vi "GenerateHistogramIndices.vi"(7 "Last laser in":bool, 11 "Laser in":bool[](array[boolean])=[FALSE, FALSE, FALSE, FALSE, FALSE, FALSE, FALSE, FALSE, FALSE, FALSE, FALSE, FALSE, FALSE, FALSE, FALSE, FALSE, FALSE, FALSE, FALSE, FALSE, FALSE, FALSE, FALSE, FALSE, FALSE, FALSE, FALSE, FALSE, FALSE, FALSE, FALSE, FALSE, FALSE, FALSE, FALSE, FALSE, FALSE, FALSE, FALSE, FALSE, FALSE, FALSE, FALSE, FALSE, FALSE, FALSE, FALSE, FALSE, FALSE, FALSE, FALSE, FALSE, FALSE, FALSE, FALSE, FALSE, FALSE, FALSE, FALSE, FALSE]) -> (3 "Index array out":i32[](array[numeric]), 5 "Last laser out":bool)   [LabVIEW 2012]
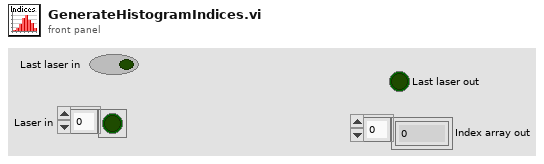
[diagram p1: front panel]
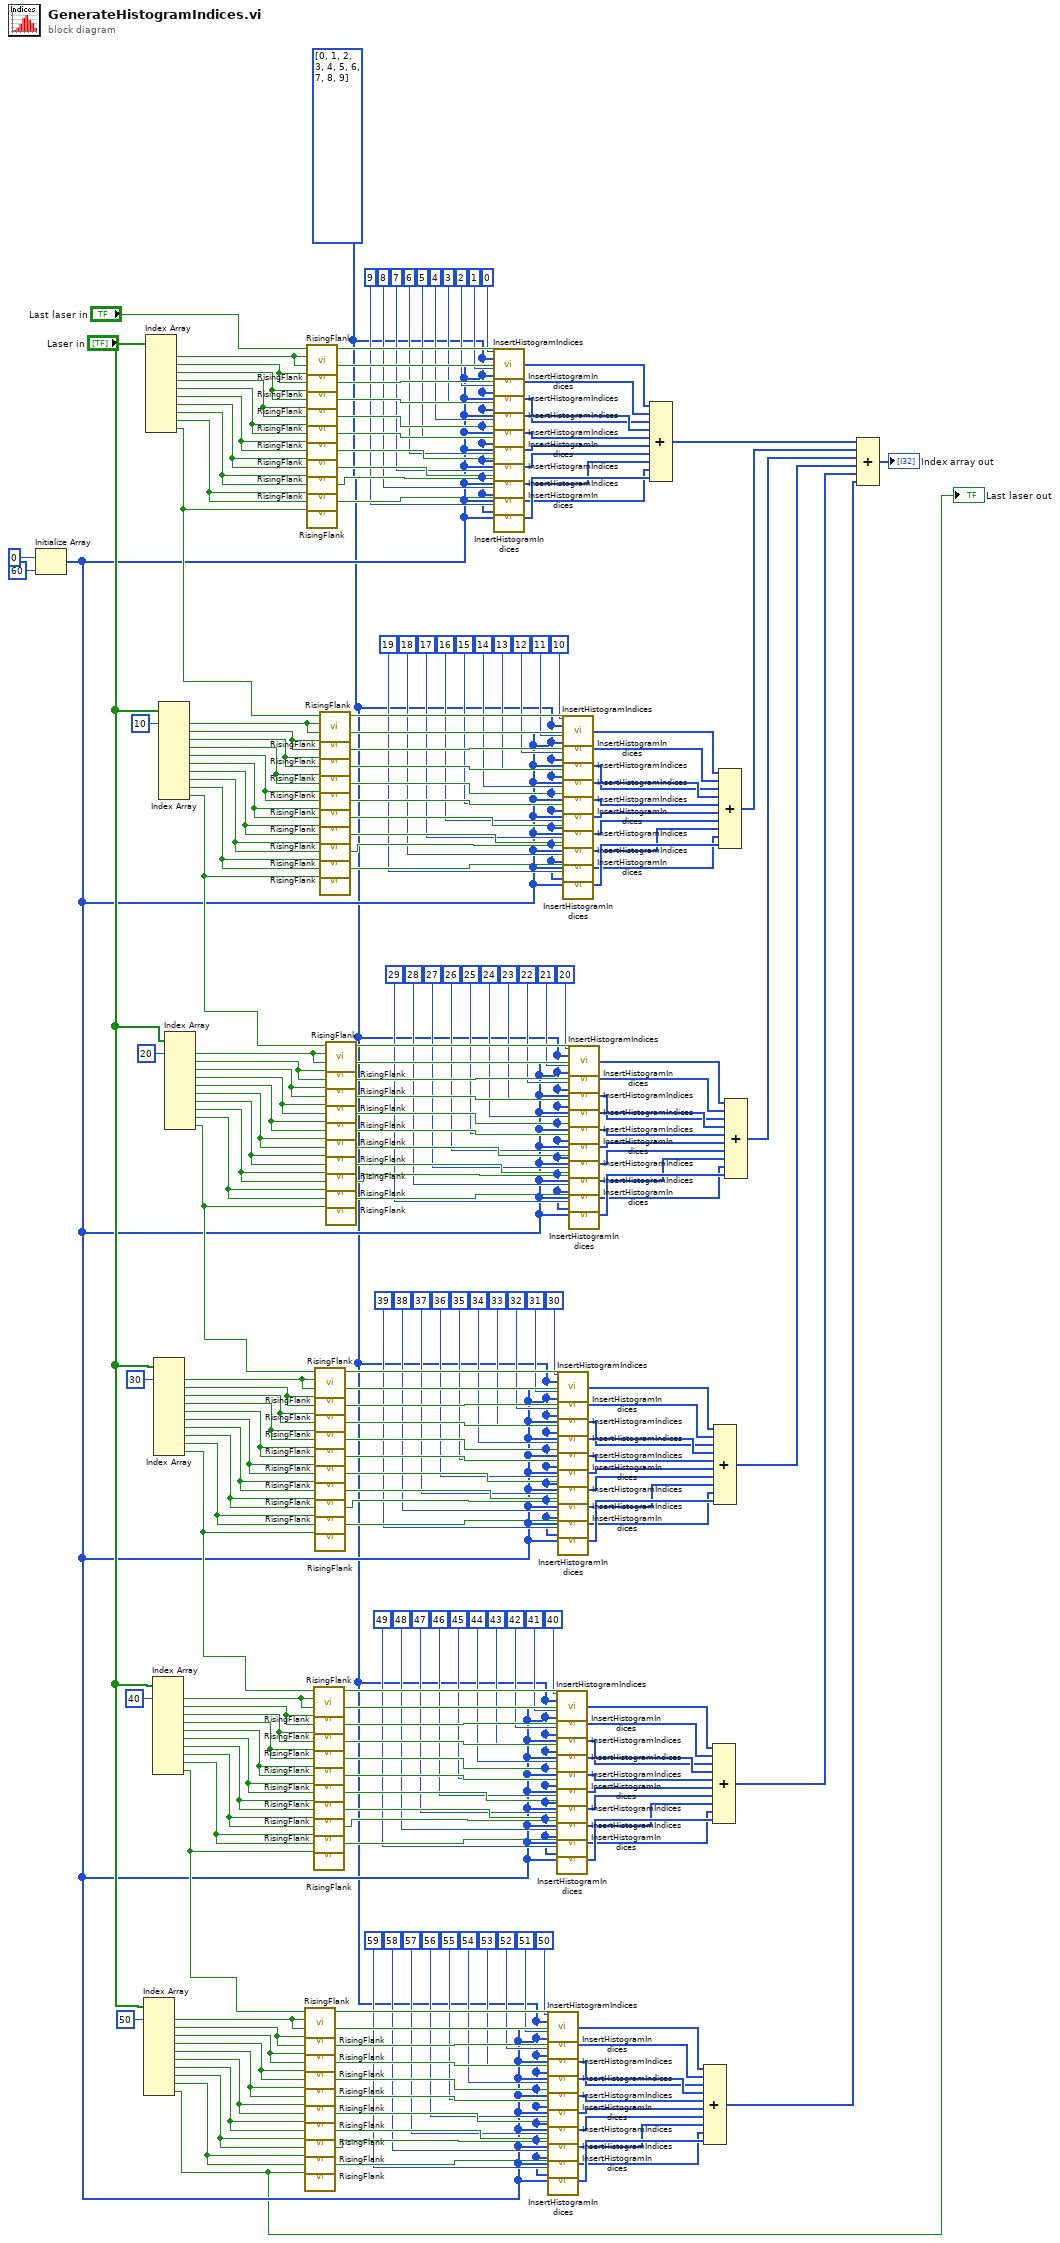
[diagram p0: block diagram]
diagram:
  w9 = i32[] [0, 1, 2, 3, 4, 5, 6, 7, 8, 9]
  n1 = Initialize Array(0, 60 ("dimension size")) -> (w10:i32[])
  n2 = Index Array(array="Laser in", index #1=50 ("index")) -> (element #1=w52:bool, element #2=w49:bool, element #3=w48:bool, element #4=w47:bool, element #5=w46:bool, element #6=w45:bool, element #7=w44:bool, element #8=w43:bool, element #9=w42:bool, element #10=w1:bool)  [unwired: 9 in]
  "Last laser out" <- w1
  n3 = Index Array(array="Laser in") -> (element #1=w255:bool, element #2=w252:bool, element #3=w251:bool, element #4=w250:bool, element #5=w249:bool, element #6=w248:bool, element #7=w247:bool, element #8=w246:bool, element #9=w245:bool, element #10=w176:bool)  [unwired: 10 in]
  n4 = Index Array(array="Laser in", index #1=40 ("index")) -> (element #1=w93:bool, element #2=w90:bool, element #3=w89:bool, element #4=w88:bool, element #5=w87:bool, element #6=w86:bool, element #7=w85:bool, element #8=w84:bool, element #9=w83:bool, element #10=w11:bool)  [unwired: 9 in]
  n5 = Index Array(array="Laser in", index #1=30 ("index")) -> (element #1=w134:bool, element #2=w131:bool, element #3=w130:bool, element #4=w129:bool, element #5=w128:bool, element #6=w127:bool, element #7=w126:bool, element #8=w125:bool, element #9=w124:bool, element #10=w53:bool)  [unwired: 9 in]
  n6 = Index Array(array="Laser in", index #1=10 ("index")) -> (element #1=w216:bool, element #2=w213:bool, element #3=w212:bool, element #4=w211:bool, element #5=w210:bool, element #6=w209:bool, element #7=w208:bool, element #8=w207:bool, element #9=w206:bool, element #10=w135:bool)  [unwired: 9 in]
  n7 = Index Array(array="Laser in", index #1=20 ("index")) -> (element #1=w175:bool, element #2=w172:bool, element #3=w171:bool, element #4=w170:bool, element #5=w169:bool, element #6=w168:bool, element #7=w167:bool, element #8=w166:bool, element #9=w165:bool, element #10=w94:bool)  [unwired: 9 in]
  n8 = call "RisingFlank.vi"("2nd sample"=w52, "1st sample"=w11) -> ("Rising flank?"=w51:bool)  [unwired: 7 in]
  n9 = call "RisingFlank.vi"("2nd sample"=w49, "1st sample"=w52) -> ("Rising flank?"=w50:bool)  [unwired: 7 in]
  n10 = call "RisingFlank.vi"("2nd sample"=w48, "1st sample"=w49) -> ("Rising flank?"=w41:bool)  [unwired: 7 in]
  n11 = call "RisingFlank.vi"("2nd sample"=w47, "1st sample"=w48) -> ("Rising flank?"=w40:bool)  [unwired: 7 in]
  n12 = call "RisingFlank.vi"("2nd sample"=w46, "1st sample"=w47) -> ("Rising flank?"=w39:bool)  [unwired: 7 in]
  n13 = call "RisingFlank.vi"("2nd sample"=w45, "1st sample"=w46) -> ("Rising flank?"=w38:bool)  [unwired: 7 in]
  n14 = call "RisingFlank.vi"("2nd sample"=w44, "1st sample"=w45) -> ("Rising flank?"=w37:bool)  [unwired: 7 in]
  n15 = call "RisingFlank.vi"("2nd sample"=w43, "1st sample"=w44) -> ("Rising flank?"=w36:bool)  [unwired: 7 in]
  n16 = call "RisingFlank.vi"("2nd sample"=w42, "1st sample"=w43) -> ("Rising flank?"=w35:bool)  [unwired: 7 in]
  n17 = call "RisingFlank.vi"("2nd sample"=w1, "1st sample"=w42) -> ("Rising flank?"=w34:bool)  [unwired: 7 in]
  n18 = call "RisingFlank.vi"("2nd sample"=w255, "1st sample"="Last laser in") -> ("Rising flank?"=w254:bool)  [unwired: 7 in]
  n19 = call "RisingFlank.vi"("2nd sample"=w252, "1st sample"=w255) -> ("Rising flank?"=w253:bool)  [unwired: 7 in]
  n20 = call "RisingFlank.vi"("2nd sample"=w251, "1st sample"=w252) -> ("Rising flank?"=w244:bool)  [unwired: 7 in]
  n21 = call "RisingFlank.vi"("2nd sample"=w250, "1st sample"=w251) -> ("Rising flank?"=w243:bool)  [unwired: 7 in]
  n22 = call "RisingFlank.vi"("2nd sample"=w249, "1st sample"=w250) -> ("Rising flank?"=w242:bool)  [unwired: 7 in]
  n23 = call "RisingFlank.vi"("2nd sample"=w248, "1st sample"=w249) -> ("Rising flank?"=w241:bool)  [unwired: 7 in]
  n24 = call "RisingFlank.vi"("2nd sample"=w247, "1st sample"=w248) -> ("Rising flank?"=w240:bool)  [unwired: 7 in]
  n25 = call "RisingFlank.vi"("2nd sample"=w246, "1st sample"=w247) -> ("Rising flank?"=w239:bool)  [unwired: 7 in]
  n26 = call "RisingFlank.vi"("2nd sample"=w245, "1st sample"=w246) -> ("Rising flank?"=w238:bool)  [unwired: 7 in]
  n27 = call "RisingFlank.vi"("2nd sample"=w176, "1st sample"=w245) -> ("Rising flank?"=w237:bool)  [unwired: 7 in]
  n28 = call "RisingFlank.vi"("2nd sample"=w93, "1st sample"=w53) -> ("Rising flank?"=w92:bool)  [unwired: 7 in]
  n29 = call "RisingFlank.vi"("2nd sample"=w90, "1st sample"=w93) -> ("Rising flank?"=w91:bool)  [unwired: 7 in]
  n30 = call "RisingFlank.vi"("2nd sample"=w89, "1st sample"=w90) -> ("Rising flank?"=w82:bool)  [unwired: 7 in]
  n31 = call "RisingFlank.vi"("2nd sample"=w88, "1st sample"=w89) -> ("Rising flank?"=w81:bool)  [unwired: 7 in]
  n32 = call "RisingFlank.vi"("2nd sample"=w87, "1st sample"=w88) -> ("Rising flank?"=w80:bool)  [unwired: 7 in]
  n33 = call "RisingFlank.vi"("2nd sample"=w86, "1st sample"=w87) -> ("Rising flank?"=w79:bool)  [unwired: 7 in]
  n34 = call "RisingFlank.vi"("2nd sample"=w85, "1st sample"=w86) -> ("Rising flank?"=w78:bool)  [unwired: 7 in]
  n35 = call "RisingFlank.vi"("2nd sample"=w84, "1st sample"=w85) -> ("Rising flank?"=w77:bool)  [unwired: 7 in]
  n36 = call "RisingFlank.vi"("2nd sample"=w83, "1st sample"=w84) -> ("Rising flank?"=w76:bool)  [unwired: 7 in]
  n37 = call "RisingFlank.vi"("2nd sample"=w11, "1st sample"=w83) -> ("Rising flank?"=w75:bool)  [unwired: 7 in]
  n38 = call "RisingFlank.vi"("2nd sample"=w134, "1st sample"=w94) -> ("Rising flank?"=w133:bool)  [unwired: 7 in]
  n39 = call "RisingFlank.vi"("2nd sample"=w131, "1st sample"=w134) -> ("Rising flank?"=w132:bool)  [unwired: 7 in]
  n40 = call "RisingFlank.vi"("2nd sample"=w130, "1st sample"=w131) -> ("Rising flank?"=w123:bool)  [unwired: 7 in]
  n41 = call "RisingFlank.vi"("2nd sample"=w129, "1st sample"=w130) -> ("Rising flank?"=w122:bool)  [unwired: 7 in]
  n42 = call "RisingFlank.vi"("2nd sample"=w128, "1st sample"=w129) -> ("Rising flank?"=w121:bool)  [unwired: 7 in]
  n43 = call "RisingFlank.vi"("2nd sample"=w127, "1st sample"=w128) -> ("Rising flank?"=w120:bool)  [unwired: 7 in]
  n44 = call "RisingFlank.vi"("2nd sample"=w126, "1st sample"=w127) -> ("Rising flank?"=w119:bool)  [unwired: 7 in]
  n45 = call "RisingFlank.vi"("2nd sample"=w125, "1st sample"=w126) -> ("Rising flank?"=w118:bool)  [unwired: 7 in]
  n46 = call "RisingFlank.vi"("2nd sample"=w124, "1st sample"=w125) -> ("Rising flank?"=w117:bool)  [unwired: 7 in]
  n47 = call "RisingFlank.vi"("2nd sample"=w53, "1st sample"=w124) -> ("Rising flank?"=w116:bool)  [unwired: 7 in]
  n48 = call "RisingFlank.vi"("2nd sample"=w216, "1st sample"=w176) -> ("Rising flank?"=w215:bool)  [unwired: 7 in]
  n49 = call "RisingFlank.vi"("2nd sample"=w213, "1st sample"=w216) -> ("Rising flank?"=w214:bool)  [unwired: 7 in]
  n50 = call "RisingFlank.vi"("2nd sample"=w212, "1st sample"=w213) -> ("Rising flank?"=w205:bool)  [unwired: 7 in]
  n51 = call "RisingFlank.vi"("2nd sample"=w211, "1st sample"=w212) -> ("Rising flank?"=w204:bool)  [unwired: 7 in]
  n52 = call "RisingFlank.vi"("2nd sample"=w210, "1st sample"=w211) -> ("Rising flank?"=w203:bool)  [unwired: 7 in]
  n53 = call "RisingFlank.vi"("2nd sample"=w209, "1st sample"=w210) -> ("Rising flank?"=w202:bool)  [unwired: 7 in]
  n54 = call "RisingFlank.vi"("2nd sample"=w208, "1st sample"=w209) -> ("Rising flank?"=w201:bool)  [unwired: 7 in]
  n55 = call "RisingFlank.vi"("2nd sample"=w207, "1st sample"=w208) -> ("Rising flank?"=w200:bool)  [unwired: 7 in]
  n56 = call "RisingFlank.vi"("2nd sample"=w206, "1st sample"=w207) -> ("Rising flank?"=w199:bool)  [unwired: 7 in]
  n57 = call "RisingFlank.vi"("2nd sample"=w135, "1st sample"=w206) -> ("Rising flank?"=w198:bool)  [unwired: 7 in]
  n58 = call "RisingFlank.vi"("2nd sample"=w175, "1st sample"=w135) -> ("Rising flank?"=w174:bool)  [unwired: 7 in]
  n59 = call "RisingFlank.vi"("2nd sample"=w172, "1st sample"=w175) -> ("Rising flank?"=w173:bool)  [unwired: 7 in]
  n60 = call "RisingFlank.vi"("2nd sample"=w171, "1st sample"=w172) -> ("Rising flank?"=w164:bool)  [unwired: 7 in]
  n61 = call "RisingFlank.vi"("2nd sample"=w170, "1st sample"=w171) -> ("Rising flank?"=w163:bool)  [unwired: 7 in]
  n62 = call "RisingFlank.vi"("2nd sample"=w169, "1st sample"=w170) -> ("Rising flank?"=w162:bool)  [unwired: 7 in]
  n63 = call "RisingFlank.vi"("2nd sample"=w168, "1st sample"=w169) -> ("Rising flank?"=w161:bool)  [unwired: 7 in]
  n64 = call "RisingFlank.vi"("2nd sample"=w167, "1st sample"=w168) -> ("Rising flank?"=w160:bool)  [unwired: 7 in]
  n65 = call "RisingFlank.vi"("2nd sample"=w166, "1st sample"=w167) -> ("Rising flank?"=w159:bool)  [unwired: 7 in]
  n66 = call "RisingFlank.vi"("2nd sample"=w165, "1st sample"=w166) -> ("Rising flank?"=w158:bool)  [unwired: 7 in]
  n67 = call "RisingFlank.vi"("2nd sample"=w94, "1st sample"=w165) -> ("Rising flank?"=w157:bool)  [unwired: 7 in]
  n68 = call "InsertHistogramIndices.vi"("Insert index"=0, "Rising flank?"=w254, "Histogram indices"=w9, "Master array in"=w10) -> ("Master array out"=w226:i32[])  [unwired: 11 in]
  n69 = call "InsertHistogramIndices.vi"("Insert index"=1, "Rising flank?"=w253, "Histogram indices"=w9, "Master array in"=w10) -> ("Master array out"=w225:i32[])  [unwired: 11 in]
  n70 = call "InsertHistogramIndices.vi"("Insert index"=2, "Rising flank?"=w244, "Histogram indices"=w9, "Master array in"=w10) -> ("Master array out"=w217:i32[])  [unwired: 11 in]
  n71 = call "InsertHistogramIndices.vi"("Insert index"=3, "Rising flank?"=w243, "Histogram indices"=w9, "Master array in"=w10) -> ("Master array out"=w218:i32[])  [unwired: 11 in]
  n72 = call "InsertHistogramIndices.vi"("Insert index"=4, "Rising flank?"=w242, "Histogram indices"=w9, "Master array in"=w10) -> ("Master array out"=w219:i32[])  [unwired: 11 in]
  n73 = call "InsertHistogramIndices.vi"("Insert index"=5, "Rising flank?"=w241, "Histogram indices"=w9, "Master array in"=w10) -> ("Master array out"=w220:i32[])  [unwired: 11 in]
  n74 = call "InsertHistogramIndices.vi"("Insert index"=6, "Rising flank?"=w240, "Histogram indices"=w9, "Master array in"=w10) -> ("Master array out"=w221:i32[])  [unwired: 11 in]
  n75 = call "InsertHistogramIndices.vi"("Insert index"=7, "Rising flank?"=w239, "Histogram indices"=w9, "Master array in"=w10) -> ("Master array out"=w222:i32[])  [unwired: 11 in]
  n76 = call "InsertHistogramIndices.vi"("Insert index"=8, "Rising flank?"=w238, "Histogram indices"=w9, "Master array in"=w10) -> ("Master array out"=w223:i32[])  [unwired: 11 in]
  n77 = call "InsertHistogramIndices.vi"("Insert index"=9, "Rising flank?"=w237, "Histogram indices"=w9, "Master array in"=w10) -> ("Master array out"=w224:i32[])  [unwired: 11 in]
  n78 = call "InsertHistogramIndices.vi"("Insert index"=50, "Rising flank?"=w51, "Histogram indices"=w9, "Master array in"=w10) -> ("Master array out"=w23:i32[])  [unwired: 11 in]
  n79 = call "InsertHistogramIndices.vi"("Insert index"=51, "Rising flank?"=w50, "Histogram indices"=w9, "Master array in"=w10) -> ("Master array out"=w22:i32[])  [unwired: 11 in]
  n80 = call "InsertHistogramIndices.vi"("Insert index"=52, "Rising flank?"=w41, "Histogram indices"=w9, "Master array in"=w10) -> ("Master array out"=w14:i32[])  [unwired: 11 in]
  n81 = call "InsertHistogramIndices.vi"("Insert index"=53, "Rising flank?"=w40, "Histogram indices"=w9, "Master array in"=w10) -> ("Master array out"=w15:i32[])  [unwired: 11 in]
  n82 = call "InsertHistogramIndices.vi"("Insert index"=54, "Rising flank?"=w39, "Histogram indices"=w9, "Master array in"=w10) -> ("Master array out"=w16:i32[])  [unwired: 11 in]
  n83 = call "InsertHistogramIndices.vi"("Insert index"=55, "Rising flank?"=w38, "Histogram indices"=w9, "Master array in"=w10) -> ("Master array out"=w17:i32[])  [unwired: 11 in]
  n84 = call "InsertHistogramIndices.vi"("Insert index"=56, "Rising flank?"=w37, "Histogram indices"=w9, "Master array in"=w10) -> ("Master array out"=w18:i32[])  [unwired: 11 in]
  n85 = call "InsertHistogramIndices.vi"("Insert index"=57, "Rising flank?"=w36, "Histogram indices"=w9, "Master array in"=w10) -> ("Master array out"=w19:i32[])  [unwired: 11 in]
  n86 = call "InsertHistogramIndices.vi"("Insert index"=58, "Rising flank?"=w35, "Histogram indices"=w9, "Master array in"=w10) -> ("Master array out"=w20:i32[])  [unwired: 11 in]
  n87 = call "InsertHistogramIndices.vi"("Insert index"=59, "Rising flank?"=w34, "Histogram indices"=w9, "Master array in"=w10) -> ("Master array out"=w21:i32[])  [unwired: 11 in]
  n88 = call "InsertHistogramIndices.vi"("Insert index"=40, "Rising flank?"=w92, "Histogram indices"=w9, "Master array in"=w10) -> ("Master array out"=w64:i32[])  [unwired: 11 in]
  n89 = call "InsertHistogramIndices.vi"("Insert index"=41, "Rising flank?"=w91, "Histogram indices"=w9, "Master array in"=w10) -> ("Master array out"=w63:i32[])  [unwired: 11 in]
  n90 = call "InsertHistogramIndices.vi"("Insert index"=42, "Rising flank?"=w82, "Histogram indices"=w9, "Master array in"=w10) -> ("Master array out"=w55:i32[])  [unwired: 11 in]
  n91 = call "InsertHistogramIndices.vi"("Insert index"=43, "Rising flank?"=w81, "Histogram indices"=w9, "Master array in"=w10) -> ("Master array out"=w56:i32[])  [unwired: 11 in]
  n92 = call "InsertHistogramIndices.vi"("Insert index"=44, "Rising flank?"=w80, "Histogram indices"=w9, "Master array in"=w10) -> ("Master array out"=w57:i32[])  [unwired: 11 in]
  n93 = call "InsertHistogramIndices.vi"("Insert index"=45, "Rising flank?"=w79, "Histogram indices"=w9, "Master array in"=w10) -> ("Master array out"=w58:i32[])  [unwired: 11 in]
  n94 = call "InsertHistogramIndices.vi"("Insert index"=46, "Rising flank?"=w78, "Histogram indices"=w9, "Master array in"=w10) -> ("Master array out"=w59:i32[])  [unwired: 11 in]
  n95 = call "InsertHistogramIndices.vi"("Insert index"=47, "Rising flank?"=w77, "Histogram indices"=w9, "Master array in"=w10) -> ("Master array out"=w60:i32[])  [unwired: 11 in]
  n96 = call "InsertHistogramIndices.vi"("Insert index"=48, "Rising flank?"=w76, "Histogram indices"=w9, "Master array in"=w10) -> ("Master array out"=w61:i32[])  [unwired: 11 in]
  n97 = call "InsertHistogramIndices.vi"("Insert index"=49, "Rising flank?"=w75, "Histogram indices"=w9, "Master array in"=w10) -> ("Master array out"=w62:i32[])  [unwired: 11 in]
  n98 = call "InsertHistogramIndices.vi"("Insert index"=30, "Rising flank?"=w133, "Histogram indices"=w9, "Master array in"=w10) -> ("Master array out"=w105:i32[])  [unwired: 11 in]
  n99 = call "InsertHistogramIndices.vi"("Insert index"=31, "Rising flank?"=w132, "Histogram indices"=w9, "Master array in"=w10) -> ("Master array out"=w104:i32[])  [unwired: 11 in]
  n100 = call "InsertHistogramIndices.vi"("Insert index"=32, "Rising flank?"=w123, "Histogram indices"=w9, "Master array in"=w10) -> ("Master array out"=w96:i32[])  [unwired: 11 in]
  n101 = call "InsertHistogramIndices.vi"("Insert index"=33, "Rising flank?"=w122, "Histogram indices"=w9, "Master array in"=w10) -> ("Master array out"=w97:i32[])  [unwired: 11 in]
  n102 = call "InsertHistogramIndices.vi"("Insert index"=34, "Rising flank?"=w121, "Histogram indices"=w9, "Master array in"=w10) -> ("Master array out"=w98:i32[])  [unwired: 11 in]
  n103 = call "InsertHistogramIndices.vi"("Insert index"=35, "Rising flank?"=w120, "Histogram indices"=w9, "Master array in"=w10) -> ("Master array out"=w99:i32[])  [unwired: 11 in]
  n104 = call "InsertHistogramIndices.vi"("Insert index"=36, "Rising flank?"=w119, "Histogram indices"=w9, "Master array in"=w10) -> ("Master array out"=w100:i32[])  [unwired: 11 in]
  n105 = call "InsertHistogramIndices.vi"("Insert index"=37, "Rising flank?"=w118, "Histogram indices"=w9, "Master array in"=w10) -> ("Master array out"=w101:i32[])  [unwired: 11 in]
  n106 = call "InsertHistogramIndices.vi"("Insert index"=38, "Rising flank?"=w117, "Histogram indices"=w9, "Master array in"=w10) -> ("Master array out"=w102:i32[])  [unwired: 11 in]
  n107 = call "InsertHistogramIndices.vi"("Insert index"=39, "Rising flank?"=w116, "Histogram indices"=w9, "Master array in"=w10) -> ("Master array out"=w103:i32[])  [unwired: 11 in]
  n108 = call "InsertHistogramIndices.vi"("Insert index"=10, "Rising flank?"=w215, "Histogram indices"=w9, "Master array in"=w10) -> ("Master array out"=w187:i32[])  [unwired: 11 in]
  n109 = call "InsertHistogramIndices.vi"("Insert index"=11, "Rising flank?"=w214, "Histogram indices"=w9, "Master array in"=w10) -> ("Master array out"=w186:i32[])  [unwired: 11 in]
  n110 = call "InsertHistogramIndices.vi"("Insert index"=12, "Rising flank?"=w205, "Histogram indices"=w9, "Master array in"=w10) -> ("Master array out"=w178:i32[])  [unwired: 11 in]
  n111 = call "InsertHistogramIndices.vi"("Insert index"=13, "Rising flank?"=w204, "Histogram indices"=w9, "Master array in"=w10) -> ("Master array out"=w179:i32[])  [unwired: 11 in]
  n112 = call "InsertHistogramIndices.vi"("Insert index"=14, "Rising flank?"=w203, "Histogram indices"=w9, "Master array in"=w10) -> ("Master array out"=w180:i32[])  [unwired: 11 in]
  n113 = call "InsertHistogramIndices.vi"("Insert index"=15, "Rising flank?"=w202, "Histogram indices"=w9, "Master array in"=w10) -> ("Master array out"=w181:i32[])  [unwired: 11 in]
  n114 = call "InsertHistogramIndices.vi"("Insert index"=16, "Rising flank?"=w201, "Histogram indices"=w9, "Master array in"=w10) -> ("Master array out"=w182:i32[])  [unwired: 11 in]
  n115 = call "InsertHistogramIndices.vi"("Insert index"=17, "Rising flank?"=w200, "Histogram indices"=w9, "Master array in"=w10) -> ("Master array out"=w183:i32[])  [unwired: 11 in]
  n116 = call "InsertHistogramIndices.vi"("Insert index"=18, "Rising flank?"=w199, "Histogram indices"=w9, "Master array in"=w10) -> ("Master array out"=w184:i32[])  [unwired: 11 in]
  n117 = call "InsertHistogramIndices.vi"("Insert index"=19, "Rising flank?"=w198, "Histogram indices"=w9, "Master array in"=w10) -> ("Master array out"=w185:i32[])  [unwired: 11 in]
  n118 = call "InsertHistogramIndices.vi"("Insert index"=20, "Rising flank?"=w174, "Histogram indices"=w9, "Master array in"=w10) -> ("Master array out"=w146:i32[])  [unwired: 11 in]
  n119 = call "InsertHistogramIndices.vi"("Insert index"=21, "Rising flank?"=w173, "Histogram indices"=w9, "Master array in"=w10) -> ("Master array out"=w145:i32[])  [unwired: 11 in]
  n120 = call "InsertHistogramIndices.vi"("Insert index"=22, "Rising flank?"=w164, "Histogram indices"=w9, "Master array in"=w10) -> ("Master array out"=w137:i32[])  [unwired: 11 in]
  n121 = call "InsertHistogramIndices.vi"("Insert index"=23, "Rising flank?"=w163, "Histogram indices"=w9, "Master array in"=w10) -> ("Master array out"=w138:i32[])  [unwired: 11 in]
  n122 = call "InsertHistogramIndices.vi"("Insert index"=24, "Rising flank?"=w162, "Histogram indices"=w9, "Master array in"=w10) -> ("Master array out"=w139:i32[])  [unwired: 11 in]
  n123 = call "InsertHistogramIndices.vi"("Insert index"=25, "Rising flank?"=w161, "Histogram indices"=w9, "Master array in"=w10) -> ("Master array out"=w140:i32[])  [unwired: 11 in]
  n124 = call "InsertHistogramIndices.vi"("Insert index"=26, "Rising flank?"=w160, "Histogram indices"=w9, "Master array in"=w10) -> ("Master array out"=w141:i32[])  [unwired: 11 in]
  n125 = call "InsertHistogramIndices.vi"("Insert index"=27, "Rising flank?"=w159, "Histogram indices"=w9, "Master array in"=w10) -> ("Master array out"=w142:i32[])  [unwired: 11 in]
  n126 = call "InsertHistogramIndices.vi"("Insert index"=28, "Rising flank?"=w158, "Histogram indices"=w9, "Master array in"=w10) -> ("Master array out"=w143:i32[])  [unwired: 11 in]
  n127 = call "InsertHistogramIndices.vi"("Insert index"=29, "Rising flank?"=w157, "Histogram indices"=w9, "Master array in"=w10) -> ("Master array out"=w144:i32[])  [unwired: 11 in]
  n128 = Compound Arithmetic op=ADD(w226, w225, w217, w218, w219, w220, w221, w222, w223, w224) -> (w8:i32[])
  n129 = Compound Arithmetic op=ADD(w23, w22, w14, w15, w16, w17, w18, w19, w20, w21) -> (w3:i32[])
  n130 = Compound Arithmetic op=ADD(w64, w63, w55, w56, w57, w58, w59, w60, w61, w62) -> (w4:i32[])
  n131 = Compound Arithmetic op=ADD(w105, w104, w96, w97, w98, w99, w100, w101, w102, w103) -> (w5:i32[])
  n132 = Compound Arithmetic op=ADD(w187, w186, w178, w179, w180, w181, w182, w183, w184, w185) -> (w7:i32[])
  n133 = Compound Arithmetic op=ADD(w146, w145, w137, w138, w139, w140, w141, w142, w143, w144) -> (w6:i32[])
  n134 = Compound Arithmetic op=ADD(w8, w7, w6, w5, w4, w3) -> (→"Index array out":i32[])
